vi "Close.vi"(8 "Error In":errorcluster, 11 "KinectSensor References":T1) -> (0 "Error Out":errorcluster)   [LabVIEW 2011, in "KinectOne.lvlib"]
doc: "Closes the current Kinect session."
uses:
  KinectOne.lvlib
  Private/Type Defs/KinectSensor References.ctl
  Microsoft.Kinect
  C:/github/makerhub/KinectOne/LabVIEW/vi.lib/MakerHub/KinectOne/Private/Libs/BodyFrameDataInterface.dll
  Private/Libs/BodyFrameDataInterface.dll
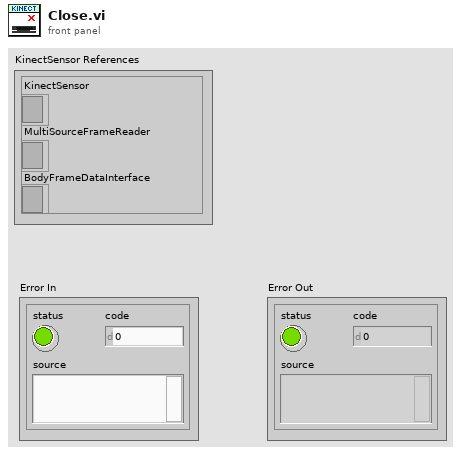
[diagram p1: front panel]
types:
  T1 = typedef "KinectOne.lvlib/KinectSensor References.ctl" = cluster{"KinectSensor":refnum<k24>, "MultiSourceFrameReader":refnum<k24>, "BodyFrameDataInterface":refnum<k24>}
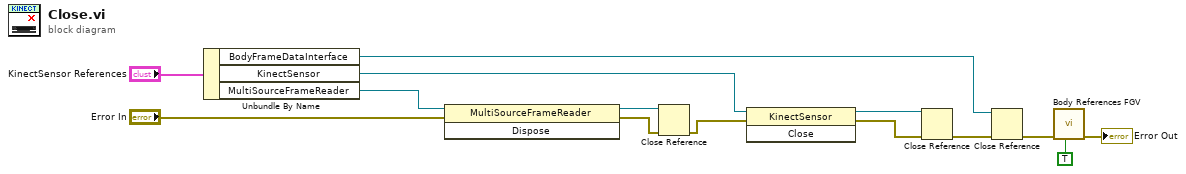
[diagram p0: block diagram]
diagram:
  n1 = Unbundle By Name("KinectSensor References") -> ("BodyFrameDataInterface"=w5:refnum<k24>, "KinectSensor"=w7:refnum<k24>, "MultiSourceFrameReader"=w8:refnum<k24>)
  n2 = invoke class="MultiSourceFrameReader" method="Dispose"(reference=w8, error in="Error In") -> (reference out=w14:refnum<k24>, error out=w13:errorcluster)  [unwired: 1 in, 1 out]
  n3 = Close Reference(reference=w14, error in (no error)=w13) -> (error out=w12:errorcluster)
  n4 = invoke class="KinectSensor" method="Close"(reference=w7, error in=w12) -> (reference out=w11:refnum<k24>, error out=w10:errorcluster)  [unwired: 1 in, 1 out]
  n5 = Close Reference(reference=w11, error in (no error)=w10) -> (error out=w6:errorcluster)
  n6 = Close Reference(reference=w5, error in (no error)=w6) -> (error out=w4:errorcluster)
  n7 = call "Body References FGV.vi"("Destroy References?"=TRUE, "error in (no error)"=w4) -> ("error out"=→"Error Out":errorcluster)  [unwired: 9 in]
